vi "BandNoise Test Settings Get Configuration Data.vi"(8 "error in (no error)":errorcluster, 10 "Configuration Name":string, 11 "Band Noise Test Settings in":refnum<class "Band Noise Test Settings.lvclass">=refnum) -> (0 "error out":errorcluster, 2 "Band Noise Test Settings":T1, 3 "Band Noise Test Settings out":refnum<class "Band Noise Test Settings.lvclass">)   [LabVIEW 2016, in "Band Noise Test Settings.lvlib" / "Band Noise Test Settings.lvclass"]
uses:
  Band Noise Test Settings.lvclass
  Controls/Band Noise Settings Cluster.ctl
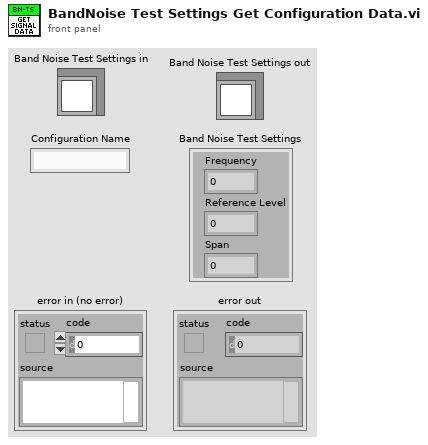
[diagram p1: front panel]
types:
  T1 = typedef "Band Noise Test Settings.lvlib/Band Noise Test Settings.lvclass/Band Noise Settings Cluster.ctl" = cluster{"Frequency":dbl, "Reference Level":dbl, "Span":dbl}
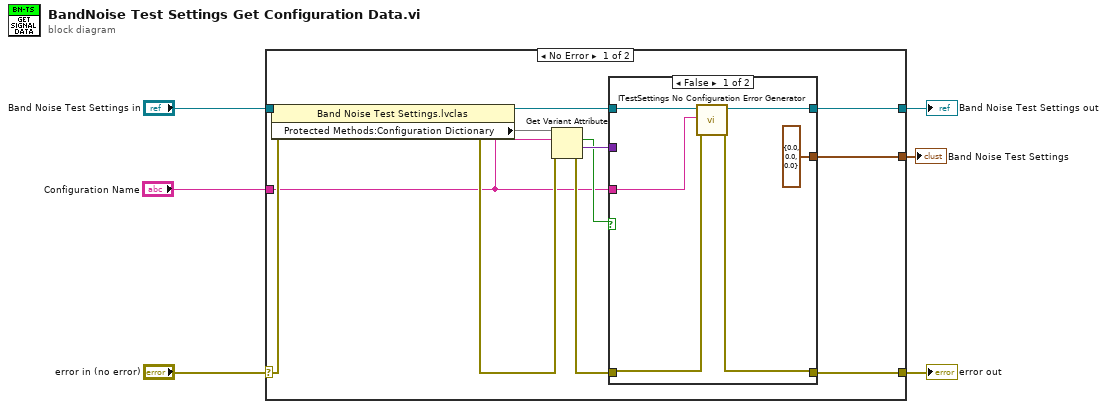
[diagram p0: block diagram]
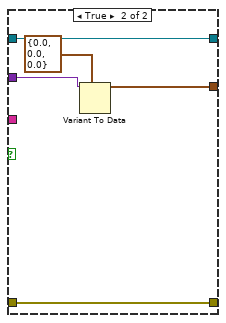
[diagram p2: hidden frame]
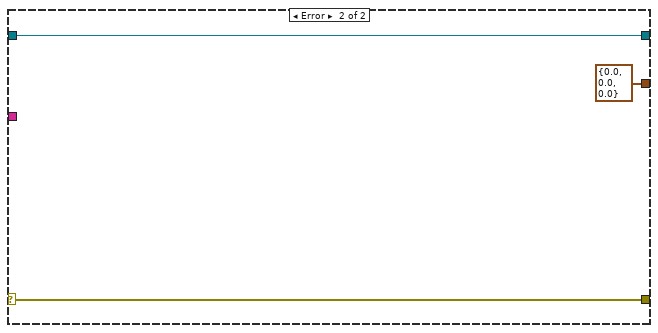
[diagram p3: hidden frame]
diagram:
  n1 = case shown="No Error" "error in (no error)" {
    selector: "error in (no error)" -> [w18 w32]
    tunnel: [w8 w32] -> w5
    tunnel: [w9 w31] -> w3
    tunnel: "Band Noise Test Settings in" -> [w17 w31]
    tunnel: "Configuration Name" -> [w7 _]
    tunnel: [w13 T1 {"Frequency"=0.0, "Reference Level"=0.0, "Span"=0.0} ("Band Noise Test Settings")] -> w1
    frame No Error {
      n2 = property class="Band Noise Test Settings.lvclas"(reference=w17, error in=w18) -> (reference out=w10:refnum<class "Band Noise Test Settings.lvclass">, error out=w15:errorcluster, "Protected Methods:Configuration Dictionary"=w16)
      n3 = Get Variant Attribute(Variant=w16, name=w7, error in=w15) -> (found=w12:bool, value=w14:variant, error out=w11:errorcluster)  [unwired: 1 in, 1 out]
      n4 = case shown="False" w12 {
        tunnel: w14 -> [_ w29]
        tunnel: [T1 {"Frequency"=0.0, "Reference Level"=0.0, "Span"=0.0} ("Band Noise Test Settings") w28] -> w13
        tunnel: w11 -> [w22 w26]
        tunnel: w10 -> [w24 w27]
        tunnel: [w23 w27] -> w9
        tunnel: [w21 w26] -> w8
        tunnel: w7 -> [w20 _]
        frame False {
          n5 = call-dynamic "ITestSettings No Configuration Error Generator.vi"("error in (no error)"=w22, "Configuration In"=w20, "ITestSettings in"=w24) -> ("error out"=w21:errorcluster, "ITestSettings out"=w23:refnum<class "Band Noise Test Settings.lvclass">)  [unwired: 7 in]
        }
        frame True {
          n6 = Variant To Data(type=T1 {"Frequency"=0.0, "Reference Level"=0.0, "Span"=0.0} ("Band Noise Test Settings"), Variant=w29) -> (data=w28:T1)  [unwired: 1 in, 1 out]
        }
      }
    }
    frame Error {
    }
  }
  "error out" <- w5
  "Band Noise Test Settings out" <- w3
  "Band Noise Test Settings" <- w1
